vi "Write Requestee.vi"(8 "error in (no error)":errorcluster, 10 "Requestee":string, 11 "Message with Names in":refnum<class "Message with Names.lvclass">) -> (0 "error out":errorcluster, 3 "Message with Names out":refnum<class "Message with Names.lvclass">)   [LabVIEW 2015, in "Message with Names.lvclass"]
uses:
  Message with Names.lvclass
  Message with Names.lvclass/Message with Names.ctl
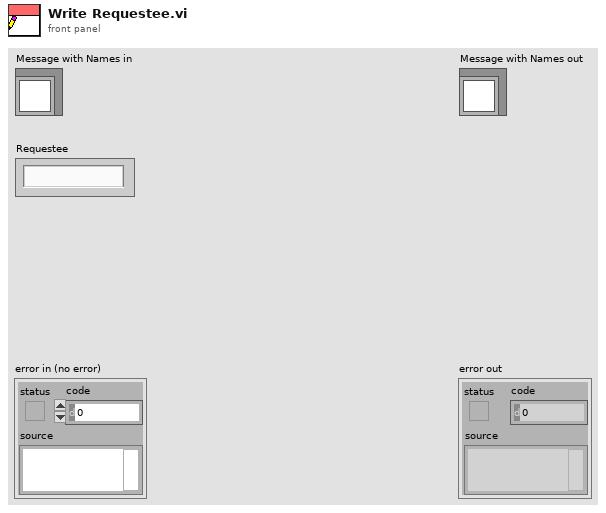
[diagram p1: front panel]
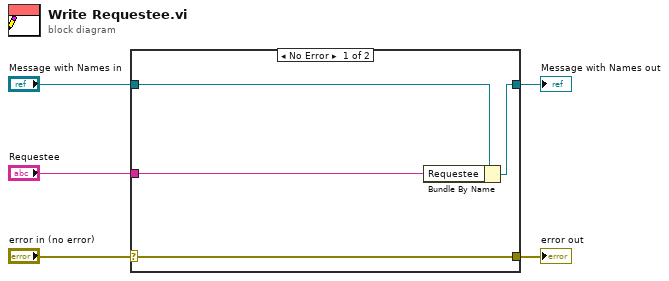
[diagram p0: block diagram]
diagram:
  n1 = case shown="No Error" "error in (no error)" {
    selector: "error in (no error)" -> [w9 w10]
    tunnel: [w9 w10] -> w4
    tunnel: [w7 w11] -> w2
    tunnel: "Message with Names in" -> [w8 w11]
    tunnel: "Requestee" -> [w6 _]
    frame No Error {
      n2 = Bundle By Name(cluster=w8, "Requestee"=w6) -> (w7:refnum<class "Message with Names.lvclass">)
    }
    frame Error {
    }
  }
  "error out" <- w4
  "Message with Names out" <- w2
